vi "UserEventDefine.vi"() -> ()   [LabVIEW 2014]
uses:
  45cb42c8-f8a3-49e2-bb66-c66450618245.vi
panel:
  out "Boolean":bool
  out "Numeric":dbl
  out "String":string
  out "UserEVTime":u32
  in  "stop":bool
  in  "Cluster":T1
  in  "Text Ring":u16(ring) items=["None", "FormA", "FormB"]
  out "Time":u32
  in  "ButtonB":bool
  in  "ButtonA":bool
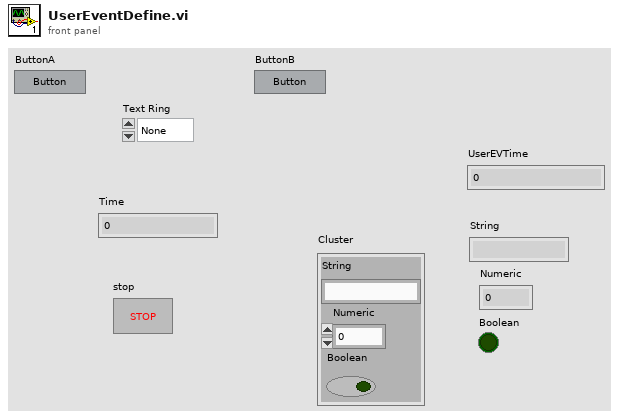
[diagram p1: front panel]
types:
  T1 = cluster{"String":string, "Numeric":dbl, "Boolean":bool}
  T2 = cluster{"type":string, "number: 0 to 1":dbl, bool}
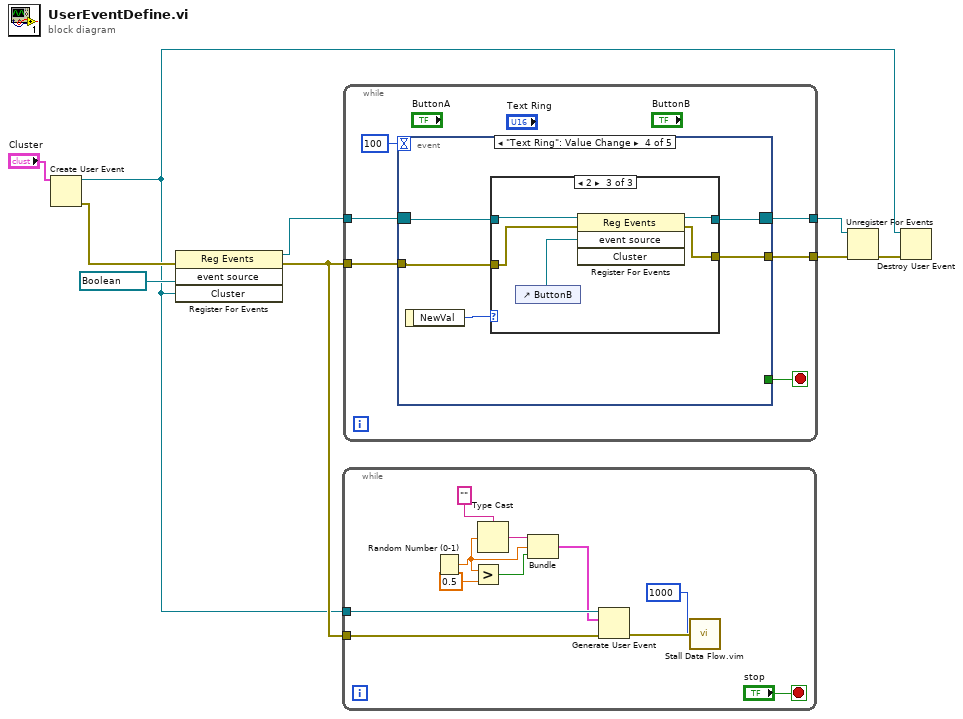
[diagram p0: block diagram]
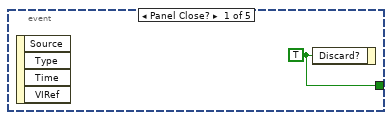
[diagram p2: hidden frame]
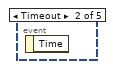
[diagram p3: hidden frame]
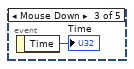
[diagram p4: hidden frame]
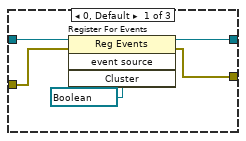
[diagram p5: hidden frame]
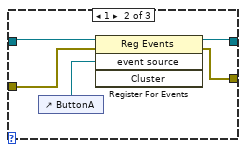
[diagram p6: hidden frame]
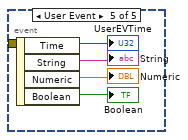
[diagram p7: hidden frame]
diagram:
  n1 = Create User Event(user event datatype="Cluster") -> (user event=w1:refnum<user-event>, error out=w4:errorcluster)  [unwired: 1 in]
  n2 = register-events(error in=w4, refnum<vi> refnum ("event source"), w1) -> (reference out=w9:refnum<event-registration>, error out=w3:errorcluster)  [unwired: 1 in]
  n3 = while {
    tunnel: w1 -> [w20]
    tunnel: w3 -> [w19]
    stop <- "stop" stop-if-true
    n4 = Random Number (0-1)() -> (number: 0 to 1=w15:dbl)
    n5 = Greater?(x=w15, y=0.5) -> (0:w14:bool)
    n6 = Type Cast(type="", x=w15) -> (*(type *) &x=w16:string)
    n7 = Bundle("type"=w16, "number: 0 to 1"=w15, w14) -> (w13:T2)  [unwired: 1 in]
    n8 = Generate User Event(user event=w20, event data cluster=w13, error in=w19) -> (error out=w11:errorcluster)  [unwired: 1 in, 1 out]
    n9 = call "Stall Data Flow.vim"("value in"=w11, "milliseconds to wait"=u32 1000) -> ()  [unwired: 2 out]
  }
  n10 = while {
    tunnel: w3 -> [w24]
    tunnel: w9 -> [w23]
    tunnel: [w22] -> w7
    tunnel: [w21] -> w6
    stop <- w25 stop-if-true
    n11 = event shown="[3] \"Text Ring\": Value Change" {
      selector: w23 -> [_ _ _ w31 _]
      dyn-events: [_ _ _ w32 _] -> w21
      timeout: 100 -> [_ _ _ _ _]
      tunnel: [w27 _ _ _ _] -> w25
      tunnel: w24 -> [_ _ _ w30 _]
      tunnel: [_ _ _ w29 _] -> w22
      event Panel Close? {
        w27 = TRUE ("Discard?")
        n12 = event-data() -> ()  [unwired: 1 in, 4 out]
        n13 = event-data("Discard?"=w27) -> ()  [unwired: 1 in, 1 out]
      }
      event Timeout {
        n14 = event-data() -> ()  [unwired: 1 in, 1 out]
      }
      event Mouse Down {
        n15 = event-data() -> ("Time"=→"Time":u32)  [unwired: 1 in]
      }
      event "Text Ring": Value Change {
        n16 = event-data() -> ("NewVal"=w33:u16)  [unwired: 1 in]
        n17 = case shown="2" w33 {
          tunnel: [w37 w42 w47] -> w32
          tunnel: w31 -> [w38 w43 w48]
          tunnel: w30 -> [w35 w40 w45]
          tunnel: [w34 w39 w44] -> w29
          frame 0, Default {
            n18 = register-events(reference=w38, error in=w35, refnum<vi> refnum ("event source")) -> (reference out=w37:refnum<event-registration>, error out=w34:errorcluster)  [unwired: 1 in]
          }
          frame 1 {
            n19 = control-ref of="ButtonA"() -> (w41:refnum<vi>)
            n20 = register-events(reference=w43, error in=w40, w41) -> (reference out=w42:refnum<event-registration>, error out=w39:errorcluster)  [unwired: 1 in]
          }
          frame 2 {
            n21 = control-ref of="ButtonB"() -> (w46:refnum<vi>)
            n22 = register-events(reference=w48, error in=w45, w46) -> (reference out=w47:refnum<event-registration>, error out=w44:errorcluster)  [unwired: 1 in]
          }
        }
      }
      event User Event {
        n23 = event-data() -> ("Time"=→"UserEVTime":u32, "String"=→"String":string, "Numeric"=→"Numeric":dbl, "Boolean"=→"Boolean":bool)  [unwired: 1 in]
      }
    }
  }
  n24 = Unregister For Events(event registration refnum=w6, error in=w7) -> (error out=w2:errorcluster)
  n25 = Destroy User Event(user event=w1, error in=w2) -> ()  [unwired: 1 out]
